vi "write_params.vi"(8 "error in (no error)":errorcluster, 10 "params":T1={"n_components"=2.0, "metric"=TRUE, "n_init"=4.0, "max_iter"=300.0, "verbose"=0.0, "eps"=0.001, "n_jobs"=1.0, "random_state"=0.0, "dissimilarity"="euclidean"}, 11 "MDS in":refnum<class "MDS.lvclass">) -> (0 "error out":errorcluster, 3 "MDS out":refnum<class "MDS.lvclass">)   [LabVIEW 2020, in "MDS.lvclass"]
uses:
  MDS.lvclass
  Controls/mds_params.ctl
  MDS.lvclass/MDS.ctl
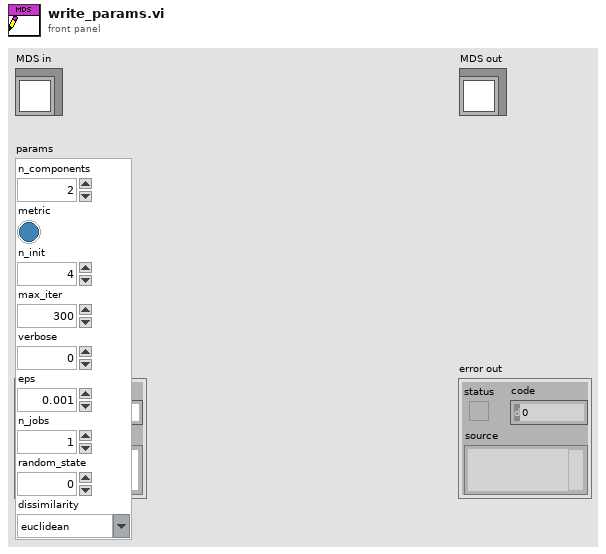
[diagram p1: front panel]
types:
  T1 = typedef "mds_params.ctl" = cluster{"n_components":dbl, "metric":bool, "n_init":dbl, "max_iter":dbl, "verbose":dbl, "eps":dbl, "n_jobs":dbl, "random_state":dbl, "dissimilarity":string}
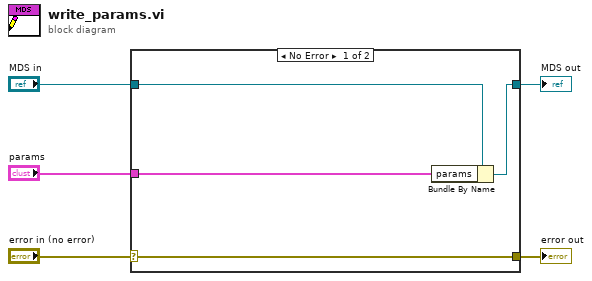
[diagram p0: block diagram]
diagram:
  n1 = case shown="No Error" "error in (no error)" {
    selector: "error in (no error)" -> [w9 w10]
    tunnel: [w9 w10] -> w4
    tunnel: [w7 w11] -> w2
    tunnel: "MDS in" -> [w8 w11]
    tunnel: "params" -> [w6 _]
    frame No Error {
      n2 = Bundle By Name(cluster=w8, "params"=w6) -> (w7:refnum<class "MDS.lvclass">)
    }
    frame Error {
    }
  }
  "error out" <- w4
  "MDS out" <- w2
